vi "Dashboard Swerve Visual.vi"(11 "Pod Setpoints (ft/s and deg)":T1) -> (2 "Robot":cluster{dbl[], dbl[]}[](array[cluster]), 3 "Pod Vectors":cluster{dbl[], dbl[]}[](array[cluster]))   [LabVIEW 2020]
uses:
  ctl/Pod Setpoints.ctl
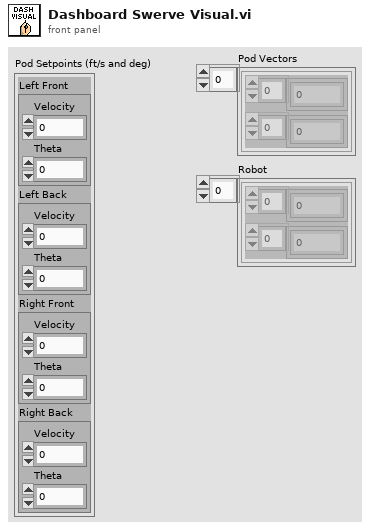
[diagram p1: front panel]
types:
  T1 = typedef "Pod Setpoints.ctl" = cluster{"Left Front":cluster{"Velocity":dbl, "Theta":dbl}, "Left Back":cluster{"Velocity":dbl, "Theta":dbl}, "Right Front":cluster{"Velocity":dbl, "Theta":dbl}, "Right Back":cluster{"Velocity":dbl, "Theta":dbl}}
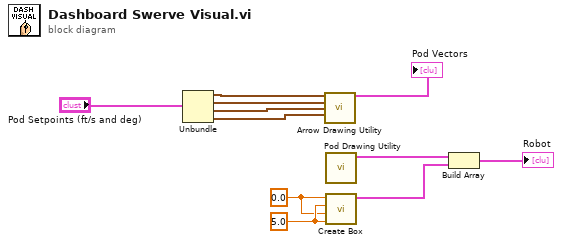
[diagram p0: block diagram]
diagram:
  w4 = 5.0 ("Right")
  w3 = 0.0 ("Left")
  n1 = Unbundle("Pod Setpoints (ft/s and deg)") -> ("Left Front"=w8:cluster{"Velocity":dbl, "Theta":dbl}, "Left Back"=w9:cluster{"Velocity":dbl, "Theta":dbl}, "Right Front"=w10:cluster{"Velocity":dbl, "Theta":dbl}, "Right Back"=w11:cluster{"Velocity":dbl, "Theta":dbl})
  n2 = call "Arrow Drawing Utility.vi"("LF Pod Setpoint"=w8, "LB Pod Setpoint"=w9, "RF Pod Setpoint"=w10, "RB Pod Setpoint"=w11) -> ("Pod Vectors"=→"Pod Vectors":cluster{dbl[], dbl[]}[])  [unwired: 9 in, 2 out]
  n3 = call "Pod Drawing Utility.vi"() -> ("Cluster"=w6:cluster{dbl[], dbl[]})  [unwired: 11 in]
  n4 = call "Create Box.vi"("Top"=w4, "Bottom"=w3, "Right"=w4, "Left"=w3) -> ("Box"=w5:cluster{dbl[], dbl[]})  [unwired: 5 in, 2 out]
  n5 = Build Array(w6, w5) -> (→"Robot":cluster{dbl[], dbl[]}[])
